vi "Parse Variant.vi"(8 "error in":errorcluster, 10 "variant":variant) -> (0 "error out":errorcluster, 1 "Types":T1(array[ring]) format="%.0x", 2 "Strings":string[](array[string]), 3 "Variants":variant[](array[variant]), 4 "Types (strings)":string[](array[string]))   [LabVIEW 2013, in "Data.PGSQL.lvclass"]
uses:
  Data.PGSQL.lvclass
  Typedefs/Errors--enum.ctl
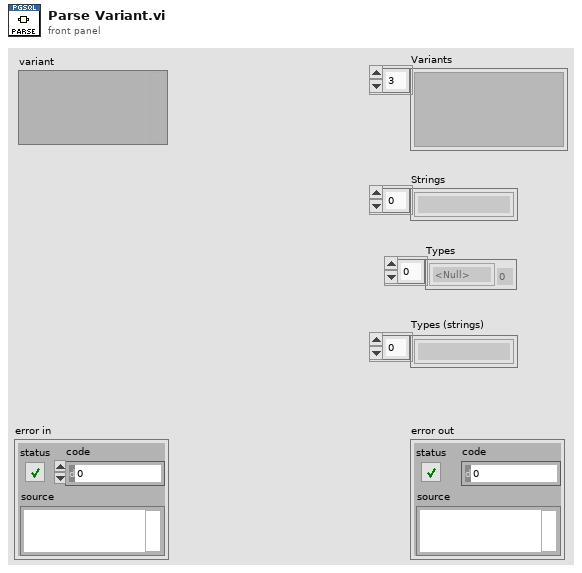
[diagram p1: front panel]
types:
  T1 = enum8{"<Null>", "I8", "I16", "I32", "I64", "U8", "U16", "U32", "U64", "SGL", "DBL", "EXT", "CSG", "CDB", "CXT", "0x0F", "0x10", "0x11", "0x12", "0x13", "0x14", "Enum U8", "Enum U16", "Enum U32", "Enum U64", "SGL PQ", "DBL PQ", "EXT PQ", "CSG PQ", "CDB PQ", "CXT PQ", "0x1F", "0x20", "Boolean", "0x22", "0x23", "0x24", "0x25", "0x26", "0x27", "0x28", "0x29", "0x2A", "0x2B", "0x2C", "0x2D", "0x2E", "0x2F", "String", "0x31", "Path", "Pict", "0x34", "0x35", "0x36", "DAQ", "0x38", "0x39", "0x3A", "0x3B", "0x3C", "0x3D", "0x3E", "0x3F", "Array", "0x41", "0x42", "0x43", "0x44", "0x45", "0x46", "0x47", "0x48", "0x49", "0x4A", "0x4B", "0x4C", "0x4D", "0x4E", "0x4F", "Cluster", "0x51", "0x52", "Variant", "Waveform", "0x55", "0x56", "0x57", "0x58", "0x59", "0x5A", "0x5B", "0x5C", "0x5D", "0x5E", "0x5F", "0x60", "0x61", "0x62", "0x63", "0x64", "0x65", "0x66", "0x67", "0x68", "0x69", "0x6A", "0x6B", "0x6C", "0x6D", "0x6E", "0x6F", "Refnum"}[]
  T2 = typedef "Data.PGSQL.lvclass/Errors--enum.ctl" = enum16{"0: None", "5005: Path Type Not Supported", "5006: Number of Variables", "5008: Cannot write two data points", "5030: Start and End Times Identical", "5031: Input is not wholly", "5033: Bad path or paths", "5040: Invalid Instrument Name", "5050: Column can only hold string", "5051 Column can only hold bool", "5052: Column can only hold double", "5053: Column can only hold int"}
  T3 = enum8{"<Null>", "I8", "I16", "I32", "I64", "U8", "U16", "U32", "U64", "SGL", "DBL", "EXT", "CSG", "CDB", "CXT", "0x0F", "0x10", "0x11", "0x12", "0x13", "0x14", "Enum U8", "Enum U16", "Enum U32", "Enum U64", "SGL PQ", "DBL PQ", "EXT PQ", "CSG PQ", "CDB PQ", "CXT PQ", "0x1F", "0x20", "Boolean", "0x22", "0x23", "0x24", "0x25", "0x26", "0x27", "0x28", "0x29", "0x2A", "0x2B", "0x2C", "0x2D", "0x2E", "0x2F", "String", "0x31", "Path", "Pict", "0x34", "0x35", "0x36", "DAQ", "0x38", "0x39", "0x3A", "0x3B", "0x3C", "0x3D", "0x3E", "0x3F", "Array", "0x41", "0x42", "0x43", "0x44", "0x45", "0x46", "0x47", "0x48", "0x49", "0x4A", "0x4B", "0x4C", "0x4D", "0x4E", "0x4F", "Cluster", "0x51", "0x52", "Variant", "Waveform", "0x55", "0x56", "0x57", "0x58", "0x59", "0x5A", "0x5B", "0x5C", "0x5D", "0x5E", "0x5F", "0x60", "0x61", "0x62", "0x63", "0x64", "0x65", "0x66", "0x67", "0x68", "0x69", "0x6A", "0x6B", "0x6C", "0x6D", "0x6E", "0x6F", "Refnum"}
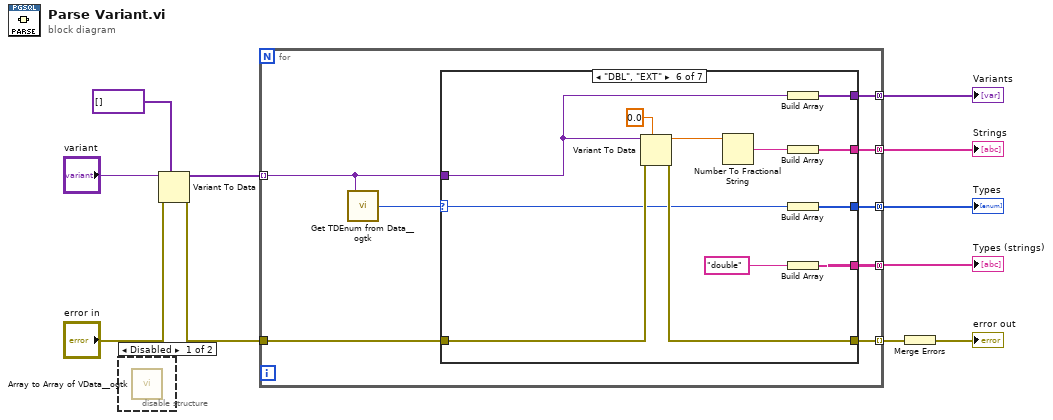
[diagram p0: block diagram]
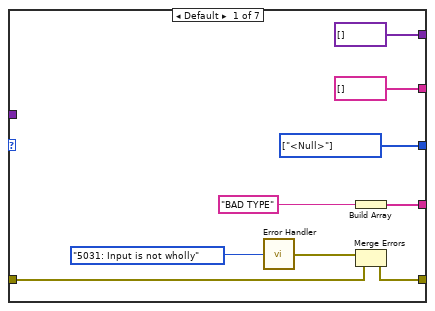
[diagram p3: hidden frame]
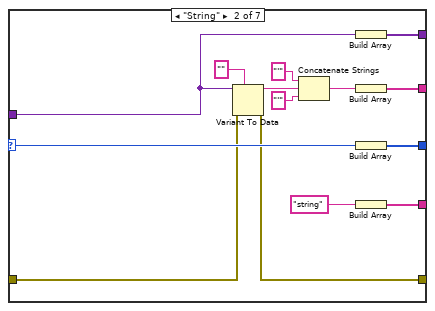
[diagram p4: hidden frame]
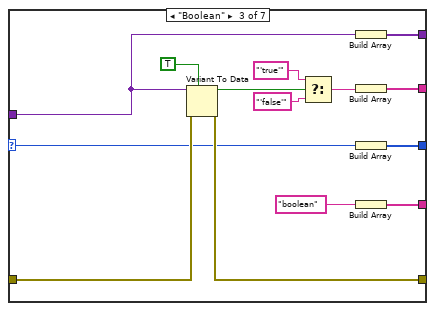
[diagram p5: hidden frame]
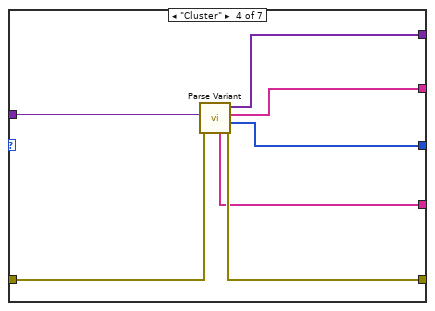
[diagram p6: hidden frame]
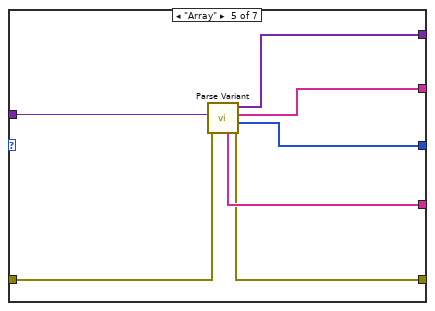
[diagram p7: hidden frame]
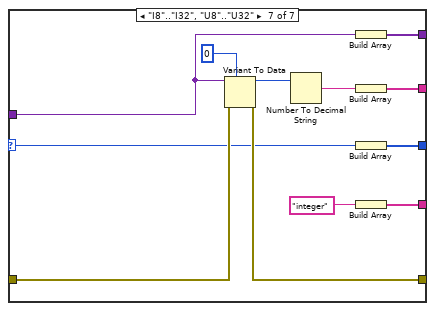
[diagram p8: hidden frame]
diagram:
  n1 = disable-structure shown="Disabled" {
    frame Disabled {
      n2 = call "Array to Array of VData__ogtk.vi"() -> ()  [unwired: 10 in, 2 out]
    }
    frame Enabled {
    }
  }
  n3 = Variant To Data(error in="error in", type=variant[] [], Variant="variant") -> (data=w2:variant[], error out=w1:errorcluster)
  n4 = for {
    tunnel: w2 -> [w14] mode=indexing
    tunnel: [w19] -> w11 mode=concatenating
    tunnel: [w18] -> w10 mode=concatenating
    tunnel: [w17] -> w9 mode=concatenating
    tunnel: [w15] -> w7 mode=indexing
    tunnel: w1 -> [w12]
    tunnel: [w16] -> w6 mode=concatenating
    n5 = call "Get TDEnum from Data__ogtk.vi"("Data"=w14) -> ("Type Descriptor Enumeration"=w13:T3)  [unwired: 4 in]
    n6 = case shown="\"DBL\", \"EXT\"" w13 {
      selector: w13 -> [_ w31 w43 _ _ w71 w83]
      tunnel: w14 -> [_ w35 w49 w63 w70 w76 w91]
      tunnel: [string[] [] ("Strings") w37 w51 w58 w69 w79 w89] -> w18
      tunnel: [w20 w36 w50 w59 w64 w80 w92] -> w19
      tunnel: [variant[] [] ("Variants") w34 w48 w57 w65 w77 w90] -> w17
      tunnel: [w26 w32 w46 w60 w68 w74 w86] -> w16
      tunnel: w12 -> [w24 w30 w45 w62 w67 w73 w85]
      tunnel: [w23 w29 w44 w61 w66 w72 w84] -> w15
      frame Default {
        w20 = T1 [enum."<Null>"] items=["<Null>", "I8", "I16", "I32", "I64", "U8", "U16", "U32", "U64", "SGL", "DBL", "EXT", "CSG", "CDB", "CXT", "0x0F", "0x10", "0x11", "0x12", "0x13", "0x14", "Enum U8", "Enum U16", "Enum U32", "Enum U64", "SGL PQ", "DBL PQ", "EXT PQ", "CSG PQ", "CDB PQ", "CXT PQ", "0x1F", "0x20", "Boolean", "0x22", "0x23", "0x24", "0x25", "0x26", "0x27", "0x28", "0x29", "0x2A", "0x2B", "0x2C", "0x2D", "0x2E", "0x2F", "String", "0x31", "Path", "Pict", "0x34", "0x35", "0x36", "DAQ", "0x38", "0x39", "0x3A", "0x3B", "0x3C", "0x3D", "0x3E", "0x3F", "Array", "0x41", "0x42", "0x43", "0x44", "0x45", "0x46", "0x47", "0x48", "0x49", "0x4A", "0x4B", "0x4C", "0x4D", "0x4E", "0x4F", "Cluster", "0x51", "0x52", "Variant", "Waveform", "0x55", "0x56", "0x57", "0x58", "0x59", "0x5A", "0x5B", "0x5C", "0x5D", "0x5E", "0x5F", "0x60", "0x61", "0x62", "0x63", "0x64", "0x65", "0x66", "0x67", "0x68", "0x69", "0x6A", "0x6B", "0x6C", "0x6D", "0x6E", "0x6F", "Refnum"] ("Types")
        n7 = call "Error Handler.vi"("Error code"=Errors--enum."5031: Input is not wholly") -> ("error out"=w21:errorcluster)
        n8 = Build Array("BAD TYPE") -> (w26:string[])
        n9 = Merge Errors(w21, w24) -> (w23:errorcluster)
      }
      frame "String" {
        n10 = Variant To Data(error in=w30, type="", Variant=w35) -> (data=w41:string, error out=w29:errorcluster)
        n11 = Concatenate Strings("'" ("string"), w41, "'" ("string")) -> (w38:string)
        n12 = Build Array(w35) -> (w34:variant[])
        n13 = Build Array(w38) -> (w37:string[])
        n14 = Build Array(w31) -> (w36:T1)
        n15 = Build Array("string") -> (w32:string[])
      }
      frame "Boolean" {
        n16 = Variant To Data(error in=w45, type=TRUE, Variant=w49) -> (data=w55:bool, error out=w44:errorcluster)
        n17 = Select(t="'true'", s=w55, f="'false'") -> (s? t:f=w52:string)
        n18 = Build Array(w49) -> (w48:variant[])
        n19 = Build Array(w52) -> (w51:string[])
        n20 = Build Array(w43) -> (w50:T1)
        n21 = Build Array("boolean") -> (w46:string[])
      }
      frame "Cluster" {
        n22 = call "Parse Variant.vi"("error in"=w62, "variant"=w63) -> ("error out"=w61:errorcluster, "Types"=w59:T1, "Strings"=w58:string[], "Variants"=w57:variant[], "Types (strings)"=w60:string[])  [unwired: 5 in]
      }
      frame "Array" {
        n23 = call "Parse Variant.vi"("error in"=w67, "variant"=w70) -> ("error out"=w66:errorcluster, "Types"=w64:T1, "Strings"=w69:string[], "Variants"=w65:variant[], "Types (strings)"=w68:string[])  [unwired: 5 in]
      }
      frame "DBL", "EXT" {
        n24 = Variant To Data(error in=w73, type=0.0, Variant=w76) -> (data=w81:dbl, error out=w72:errorcluster)
        n25 = Number To Fractional String(number=w81) -> (F-format string=w78:string)  [unwired: 3 in]
        n26 = Build Array(w76) -> (w77:variant[])
        n27 = Build Array(w78) -> (w79:string[])
        n28 = Build Array(w71) -> (w80:T1)
        n29 = Build Array("double") -> (w74:string[])
      }
      frame "I8".."I32", "U8".."U32" {
        n30 = Variant To Data(error in=w85, type=0, Variant=w91) -> (data=w93:i32, error out=w84:errorcluster)
        n31 = Number To Decimal String(number=w93) -> (decimal integer string=w88:string)  [unwired: 1 in]
        n32 = Build Array(w91) -> (w90:variant[])
        n33 = Build Array(w88) -> (w89:string[])
        n34 = Build Array(w83) -> (w92:T1)
        n35 = Build Array("integer") -> (w86:string[])
      }
    }
  }
  "Variants" <- w9
  "Types" <- w11
  "Strings" <- w10
  "Types (strings)" <- w6
  n36 = Merge Errors(w7) -> (→"error out":errorcluster)
